vi "NewPort_PM_Cmd.vi"(8 "Error In":errorcluster, 9 "USB Address":i32=1 min=1 max=15 step=1, 11 "ID Query":string="*IDN?") -> (0 "Error":errorcluster, 3 "Query Response":string)   [LabVIEW 2017]
panel:
  in  "Query\nSelect":bool
  in  "Power Reading Query":string="PM:CHANnel 1;PM:P?"
  # "ID"
  # "Power"
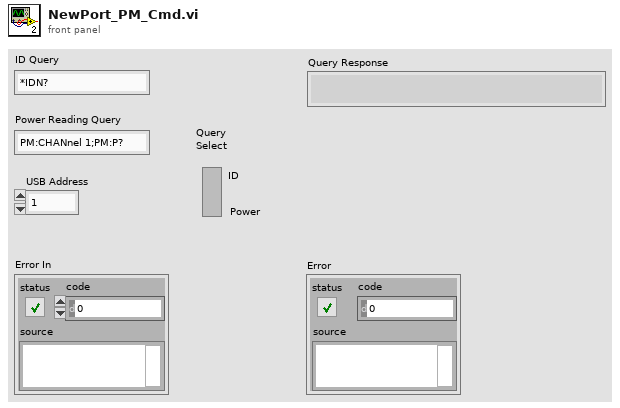
[diagram p1: front panel]
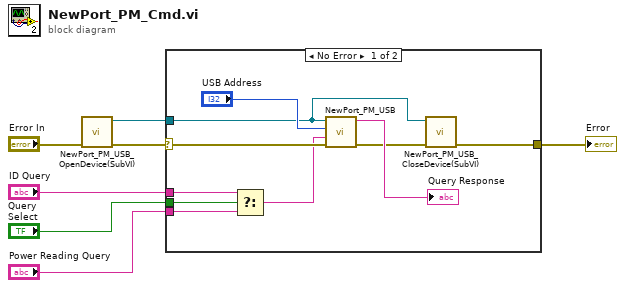
[diagram p0: block diagram]
diagram:
  n1 = call "NewPort_PM_USB_OpenDevice(SubVI).vi"("error in"="Error In") -> ("error out"=w7:errorcluster, "reference Out"=w5:refnum<k24>)  [unwired: 9 in]
  n2 = case shown="No Error" w7 {
    selector: w7 -> [w17 w18]
    tunnel: [w13 w18] -> w6
    tunnel: w5 -> [w15 _]
    tunnel: "ID Query" -> [w11 _]
    tunnel: "Query\nSelect" -> [w10 _]
    tunnel: "Power Reading Query" -> [w9 _]
    frame No Error {
      n3 = Select(t=w11, s=w10, f=w9) -> (s? t:f=w8:string)
      n4 = call "NewPort_PM_USB.vi"("error in"=w17, "PM:CMD_QUERY In"=w8, "USB Address"="USB Address", "reference"=w15) -> ("error out"=w12:errorcluster, "Query-String\nfrom Read Buffer\nComplete Info"=→"Query Response":string)  [unwired: 5 in, 1 out]
      n5 = call "NewPort_PM_USB_CloseDevice(SubVI).vi"("error in"=w12, "reference In"=w15) -> ("error out"=w13:errorcluster)  [unwired: 9 in]
    }
    frame Error {
    }
  }
  "Error" <- w6
